vi "testVi1.vi"() -> ()   [LabVIEW 2021]
panel:
  out "Output":dbl
  in  "V2":dbl
  in  "V1":dbl
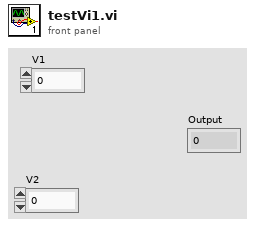
[diagram p1: front panel]
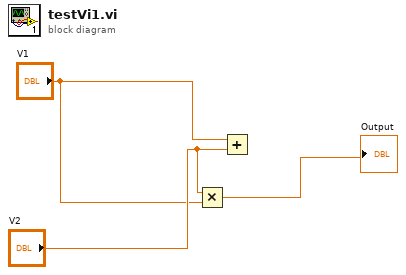
[diagram p0: block diagram]
diagram:
  n1 = Multiply(x="V2", y="V1") -> (x*y=→"Output":dbl)
  n2 = Add(x="V1", y="V2") -> ()  [unwired: 1 out]
